vi "TIM.vi"(0 "System no.":i32=1 min=1 max=4 step=1, 2 "Without parameter?":bool, 3 "Timer value":dbl=1.0 min=0.0 max=20.0 step=1.0 format="%_6g", 4 "No.of digits":i16=4, 5 "error in":errorcluster) -> (14 "Controller error":bool, 19 "error out":errorcluster)   [LabVIEW 2020]
doc: "Sets the milliseconds timer to a given value. Number of digits is the number of digits after the decimal point in the Timer value that will be sent. Without parameter the timer is resetted to zero. Controller error is TRUE if selected system reports error code is not 0.\n\nC-867, C-884:"
panel:
  # "Sets the milliseconds timer to a given value. Without \nparameter the timer is resetted to zero."
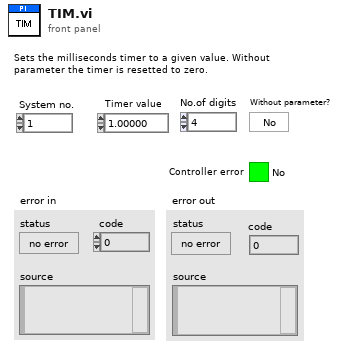
[diagram p1: front panel]
types:
  T1 = enum16{"Disable error check", "Force error check", "Use global settings"}
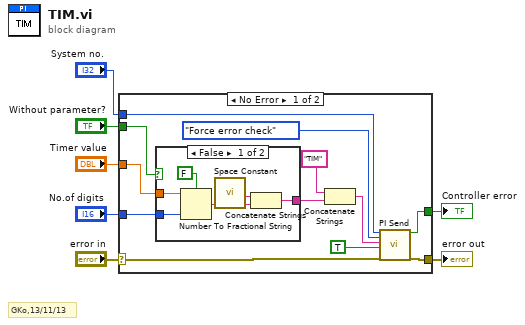
[diagram p0: block diagram]
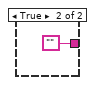
[diagram p2: hidden frame]
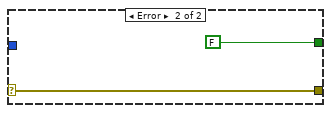
[diagram p3: hidden frame]
diagram:
  # "GKo,13/11/13"
  n1 = case shown="No Error" "error in" {
    selector: "error in" -> [w8 w28]
    tunnel: "System no." -> [w17 _]
    tunnel: "Without parameter?" -> [w14 _]
    tunnel: "No.of digits" -> [w13 _]
    tunnel: "Timer value" -> [w12 _]
    tunnel: [w10 w28] -> w3
    tunnel: [w9 FALSE ("Controller error")] -> w2
    frame No Error {
      n2 = case shown="False" w14 {
        tunnel: [w24 ""] -> w15
        tunnel: w13 -> [w23 _]
        tunnel: w12 -> [w22 _]
        frame False {
          n3 = Number To Fractional String(use system decimal point (T)=FALSE, number=w22, precision (6)=w23) -> (F-format string=w21:string)  [unwired: 1 out]
          n4 = call <vilib>:"Space Constant.vi"() -> ("String"=w25:string)
          n5 = Concatenate Strings(w25, w21) -> (w24:string)
        }
        frame True {
        }
      }
      n6 = Concatenate Strings("TIM", w15) -> (w16:string)
      n7 = call "PI Send.vi"("System no."=w17, "Error check settings"=T1."Force error check", "String to send"=w16, "Attach termination char.?"=TRUE ("Attach Linefeed?"), "error in"=w8) -> ("Controller error"=w9:bool, "error out"=w10:errorcluster)  [unwired: 1 in, 12 out]
    }
    frame Error {
    }
  }
  "error out" <- w3
  "Controller error" <- w2
